vi "_Test Modified Sync Filter.vi"() -> ()   [LabVIEW 2021, in "Math.lvlib"]
uses:
  Math.lvlib
  <vilib>/Analysis/3filter.llb/Savitzky-Golay Filter (DBL).vi
  <vilib>/Analysis/NI_AALBase.lvlib
panel:
  in  "Repeats":i32=10
  in  "Fractional Damping":dbl=0.4
  in  "Fractional Threshold":dbl=0.1
  in  "order  (3)":i32=3
  in  "side points (6)":i32=6
  in  "Array in":dbl[](array[numeric])
  out "Waveform Graph":dbl[][](graph)
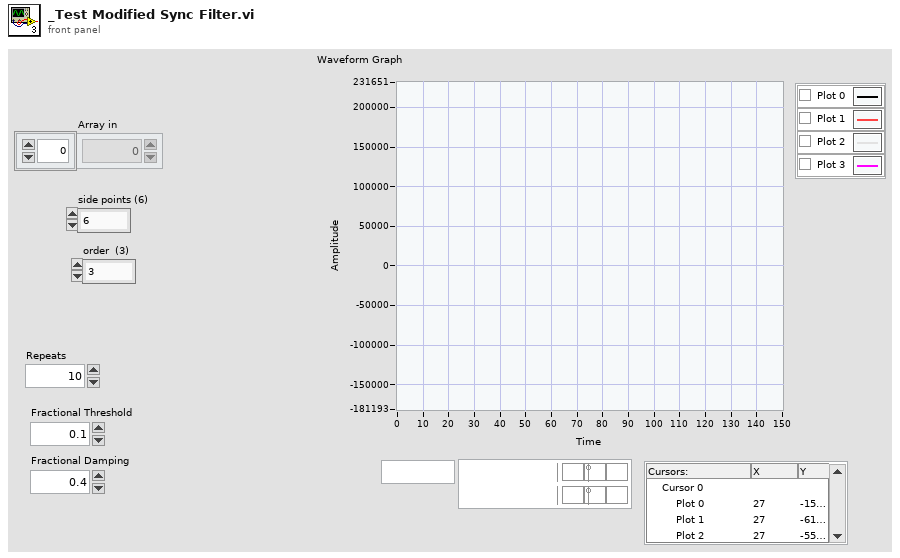
[diagram p1: front panel]
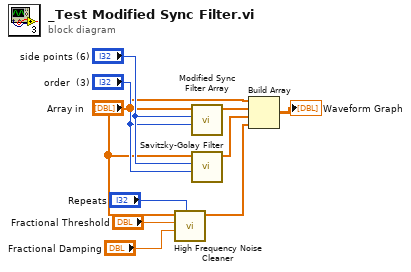
[diagram p0: block diagram]
diagram:
  n1 = call "High Frequency Noise Cleaner.vi"("Repeats"="Repeats", "Fractional Damping"="Fractional Damping", "Fractional Threshold"="Fractional Threshold", "Array in"="Array in") -> ("Array out"=w4:dbl[])  [unwired: 6 in, 1 out]
  n2 = call "Modified Sync Filter Array.vi"("order  (3)"="order  (3)", "side points (6)"="side points (6)", "Array"="Array in") -> ("Filtered Array"=w10:dbl[])  [unwired: 7 in, 1 out]
  n3 = call-poly <vilib>:"Savitzky-Golay Filter.vi"("polynomial order"="order  (3)", "side points"="side points (6)", "X"="Array in") -> ("Filtered X"=w6:dbl[])  [unwired: 7 in, 1 out]
  n4 = Build Array("Array in", w10, w6, w4) -> (→"Waveform Graph":dbl[][])
